vi "Array String Contains.vi"(3 "Regular expression":string="STOP", 4 "Case Sensitive?":bool, 5 "Array - String":string[](array[string])) -> (1 "Found?":bool, 2 "Matched String":string)   [LabVIEW 2016]
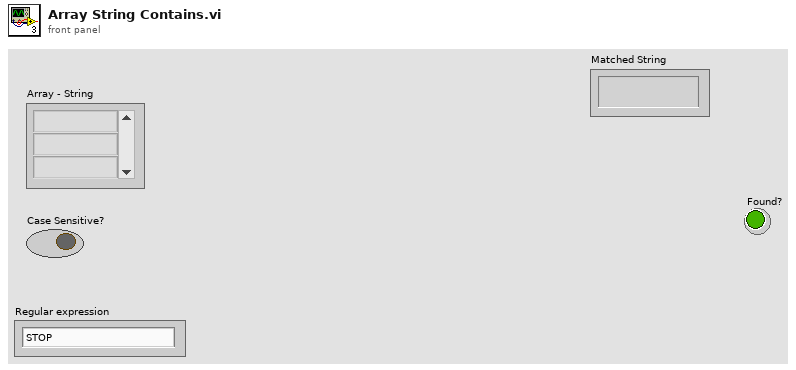
[diagram p1: front panel]
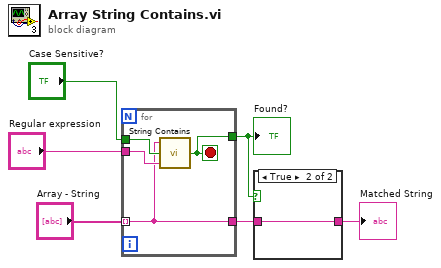
[diagram p0: block diagram]
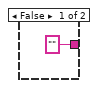
[diagram p2: hidden frame]
diagram:
  n1 = for {
    tunnel: "Array - String" -> [w7] mode=indexing
    tunnel: "Case Sensitive?" -> [w10]
    tunnel: "Regular expression" -> [w9]
    tunnel: [w8] -> w3
    tunnel: [w7] -> w1
    stop <- w8 stop-if-true
    n2 = call "String Contains.vi"("Regular expression"=w9, "Case Sensitive?"=w10, "Input String"=w7) -> ("Found?"=w8:bool)  [unwired: 1 in, 1 out]
  }
  "Found?" <- w3
  n3 = case shown="True" w3 {
    tunnel: ["" ("Input String") w12] -> w2
    tunnel: w1 -> [_ w12]
    frame False {
    }
    frame True {
    }
  }
  "Matched String" <- w2
